vi "GetArrayDataFromAcc.vi"(10 "AvgCount_powerOf2":i16, 11 "Refnum in":refnum<k21>) -> (3 "Numeric":u64)   [LabVIEW 2020]
uses:
  <vilib>/rvi/DataTransferAndStorage/Container/Common/niFpgaContainerExecOnDevCompGetState.vi
  <vilib>/rvi/Emulation/niFpgaEmulationIsFPGAContextNoSignature.vi
  <vilib>/rvi/Emulation/niFpgaSctlEmulationGetInTimedLoop.vi
  <vilib>/rvi/errors/niFpgaSetErrorForExecOnDevCompSimple.vi
  <vilib>/rvi/eio/common/nirviEmuReportErrorAndStop.vi
  <vilib>/rvi/DataTransferAndStorage/Container/Common/niFpgaContainerGetUniqueNameForEmu.vi
  <vilib>/rvi/FIFO/Fifo_Resource/nirvififoEmulationSetSize.vi
  <vilib>/rvi/FIFO/Fifo_Resource/nirviFifoEmulationQueueMgr.vi
  <instcachedir>/0/nirviFifoEmulationQueueMgr_E5CAEC123FF24DC58D834DCA3CDAA9B5.lvgen/nirviFifoEmulationQueueMgr_E5CAEC123FF24DC58D834DCA3CDAA9B5_003.vi
  <vilib>/rvi/FIFO/Fifo_Resource/nirvififoEmulationDetermineInputValidOut.vi
  <vilib>/rvi/FIFO/Fifo_Resource/nirvififoEmulationCreateLock.vi
  <vilib>/rvi/Emulation/niFpgaProcessEmulError.vi
  <vilib>/rvi/FIFO/Fifo_Resource/nirvififoEmulationObtainLock.vi
  <vilib>/rvi/FIFO/Fifo_Resource/nirvififoEmulationReleaseLock.vi
  <vilib>/rvi/occurrence/nirviWaitOnOccurrenceBase.vi
  <vilib>/rvi/errors/nirviReportUnexpectedCaseInternalError.vi
  <vilib>/rvi/errors/nirviReportUnexpectedCaseInternalError (U32).vi
  <vilib>/Utility/error.llb/Clear Errors.vi
  <vilib>/rvi/interface/RandomDataEmulation/niFpgaRandomDataHandleErrors.vi
  <vilib>/rvi/DataTransferAndStorage/Container/XNode/niFpgaContainer.xnode
  <vilib>/rvi/FIFO/Fifo_Resource/niFpgaFifoEmulationRefIn.vi
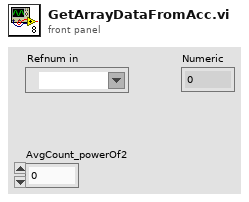
[diagram p1: front panel]
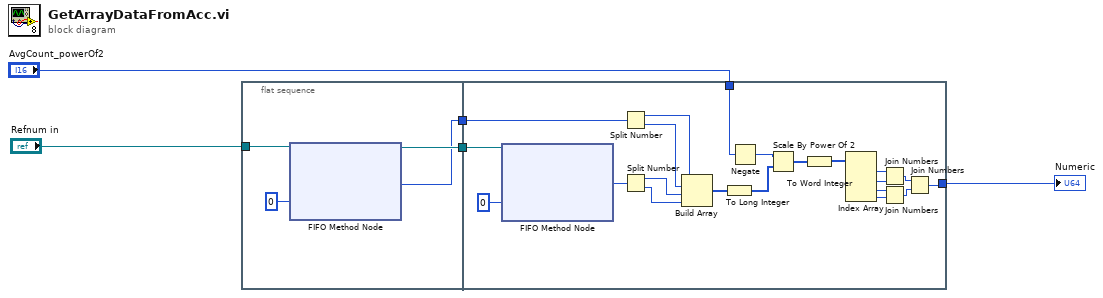
[diagram p0: block diagram]
diagram:
  n1 = flat-sequence {
    tunnel: [w8] -> w5
    tunnel: [w7] -> w4
    tunnel: "Refnum in" -> [w6]
    tunnel: w5 -> [w29]
    tunnel: w4 -> [w26]
    tunnel: [w16] -> w1
    tunnel: "AvgCount_powerOf2" -> [w15]
    frame #0 {
      n2 = xnode ("FIFO Method Node")("Timeout"=0, "FIFO In"=w6) -> ("Element"=w7:u64, "FIFO Out"=w8:refnum<k21>)  [unwired: 1 out]
    }
    frame #1 {
      n3 = xnode ("FIFO Method Node")("Timeout"=0, "FIFO In"=w29) -> ("Element"=w27:u64)  [unwired: 2 out]
      n4 = Split Number(x=w26) -> (hi(x)=w14:u32, lo(x)=w13:u32)
      n5 = Split Number(x=w27) -> (hi(x)=w12:u32, lo(x)=w11:u32)
      n6 = Build Array(w14, w13, w12, w11) -> (w10:u32[])
      n7 = To Long Integer(number=w10) -> (32bit integer=w25:i32[])
      n8 = Negate(x=w15) -> (-x=w28:i16)
      n9 = Scale By Power Of 2(n=w28, x=w25) -> (x*2^n=w24:i32[])
      n10 = To Word Integer(number=w24) -> (16bit integer=w19:i16[])
      n11 = Index Array(array=w19) -> (element #1=w20:i16, element #2=w21:i16, element #3=w22:i16, element #4=w23:i16)  [unwired: 4 in]
      n12 = Join Numbers(hi=w20, lo=w21) -> ((hi.lo)=w18:u32)
      n13 = Join Numbers(hi=w22, lo=w23) -> ((hi.lo)=w17:u32)
      n14 = Join Numbers(hi=w18, lo=w17) -> ((hi.lo)=w16:u64)
    }
  }
  "Numeric" <- w1
